vi "init.vi"(8 "error in (no error)":errorcluster, 10 "Variant":variant, 11 "generic-temp-sensor in":refnum<class "generic-temp-sensor.lvclass">) -> (0 "error out":errorcluster, 3 "generic-temp-sensor out":refnum<class "generic-temp-sensor.lvclass">)   [LabVIEW 2025, in "Temperature Sensor.lvlib" / "generic-temp-sensor.lvclass"]
uses:
  generic-temp-sensor.lvclass
  generic-temp-sensor.lvclass/generic-temp-sensor.ctl
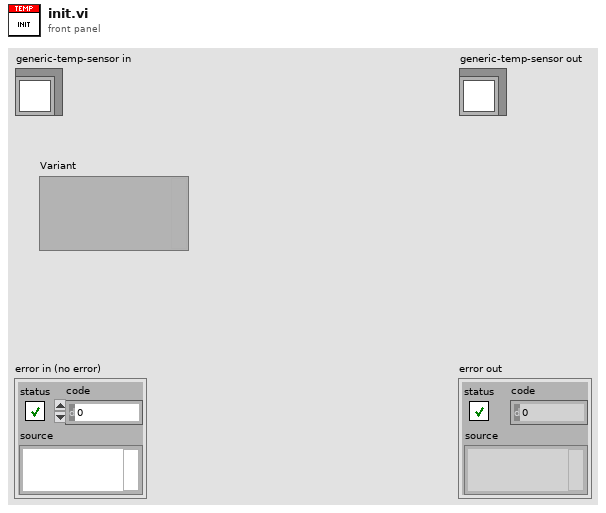
[diagram p1: front panel]
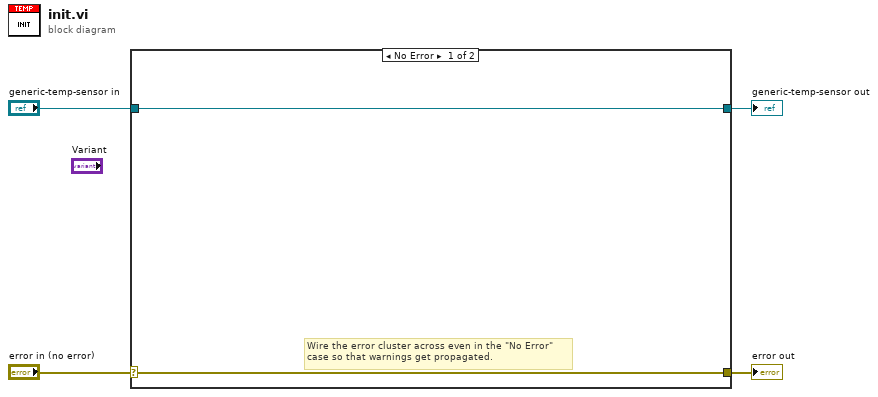
[diagram p0: block diagram]
diagram:
  n1 = case shown="No Error" "error in (no error)" {
    selector: "error in (no error)" -> [w5 w8]
    tunnel: [w5 w8] -> w3
    tunnel: [w6 w7] -> w1
    tunnel: "generic-temp-sensor in" -> [w6 w7]
    frame No Error {
      # "Wire the error cluster across even in the \"No Error\"\ncase so that warnings get propagated."
    }
    frame Error {
    }
  }
  "error out" <- w3
  "generic-temp-sensor out" <- w1
